vi "ConvertDataToNumeric.vi"(8 "error in (no error)":errorcluster, 10 "BoardType":u32, 11 "Data":u32) -> (0 "error out":errorcluster, 3 "ConvertedTime":dbl)   [LabVIEW 2022 SP3, in "EClib functions.lvlib"]
doc: "This VI supplies information on the selected channel."
uses:
  EClib functions.lvlib
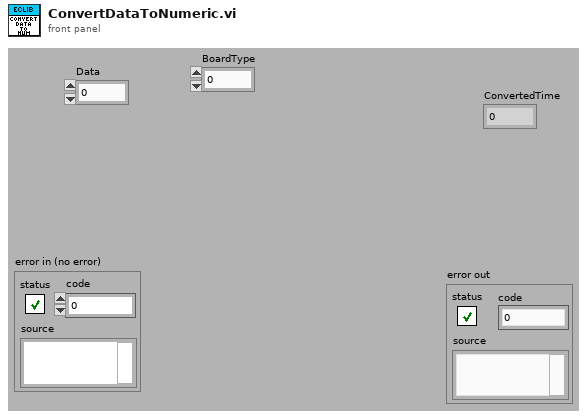
[diagram p1: front panel]
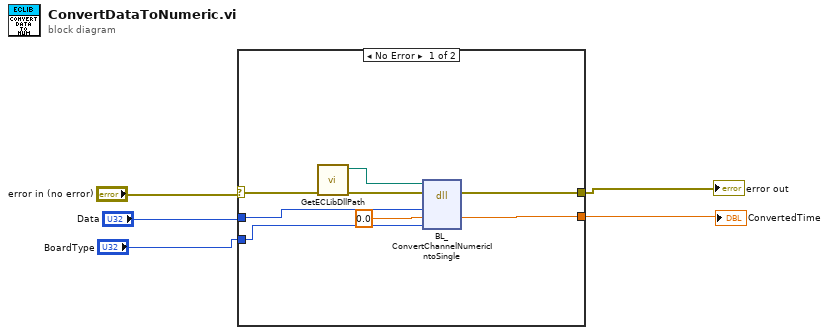
[diagram p0: block diagram]
diagram:
  n1 = case shown="No Error" "error in (no error)" {
    selector: "error in (no error)" -> [w13 w14]
    tunnel: [w7 w14] -> w2
    tunnel: "Data" -> [w12 _]
    tunnel: "BoardType" -> [w10 _]
    tunnel: [w6 _] -> w1
    frame No Error {
      n2 = call "GetECLibDllPath.vi"("error in (no error)"=w13) -> ("error out"=w9:errorcluster, "ECLibDLLPath"=w8:path)  [unwired: 9 in]
      n3 = dll-call lib="?" fn="BL_ConvertChannelNumericIntoSingle" label="ConvertNumeric"(path in=w8, error in=w9, "num"=w12, "pRetFloat"=sgl 0.0, "ChannelType"=w10) -> (error out=w7:errorcluster, "pRetFloat"=w6:sgl)  [unwired: 4 in, 1 out]
    }
    frame Error {
    }
  }
  "error out" <- w2
  "ConvertedTime" <- w1
